vi "UIRef.vi"(8 "error in":errorcluster, 11 "Modbus Slave editor node in":refnum<class "Modbus Module editor node.lvclass">) -> (0 "error out":errorcluster, 2 "VI refnum":refnum<vi>, 3 "Modbus Slave editor node out":refnum<class "Modbus Module editor node.lvclass">)   [LabVIEW 2015, in "Modbus Module editor node.lvclass"]
doc: "Platypus Framework 1.0.1.65\nNI Systems Engineering - National Instruments"
uses:
  Modbus Module editor node.lvclass
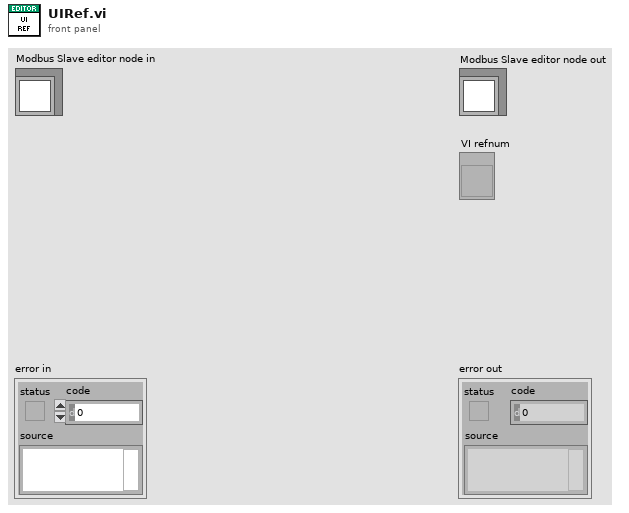
[diagram p1: front panel]
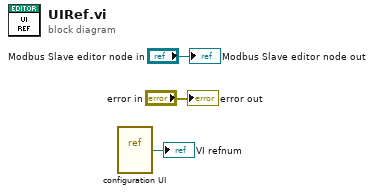
[diagram p0: block diagram]
diagram:
  n1 = vi-ref "configuration UI.vi"() -> (→"VI refnum":refnum<vi>)
  "error out" <- "error in"
  "Modbus Slave editor node out" <- "Modbus Slave editor node in"
